vi "LoadWaferImg.vi"(8 "error in (no error)":errorcluster, 11 "FrontPanelData.lvclass":refnum<class "EpiWrapper.lvclass">) -> (0 "error out":errorcluster, 3 "FrontPanelData out":refnum<class "EpiWrapper.lvclass">)   [LabVIEW 2012]
uses:
  Classes/EpiWrapper.lvclass
  Controls/Waferimage.ctl
  Classes/EpiWrapper.lvclass/EpiWrapper.ctl
  Classes/Get_WaferImg.vi
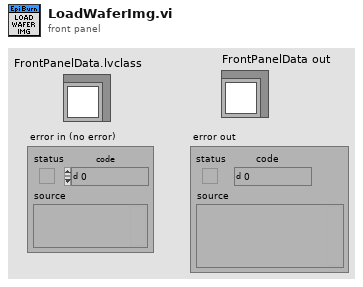
[diagram p1: front panel]
types:
  T1 = typedef "Waferimage.ctl" = picture
  T2 = typedef "LVBoundsTypeDef.ctl" = cluster{"Width":u32, "Height":u32}
  T3 = typedef "imagedata.ctl" = cluster{"image type":i32, "image depth":i32, "image":u8[], "mask":u8[], "colors":u32[], "Rectangle":cluster{"left":i16, "top":i16, "right":i16, "bottom":i16}}
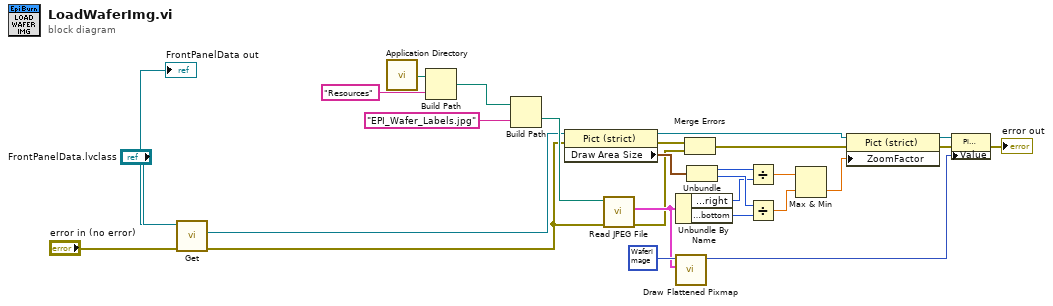
[diagram p0: block diagram]
diagram:
  n1 = call-poly "Get.vi"("error in (no error)"="error in (no error)", "FrontPanelData in"="FrontPanelData.lvclass") -> ("error out"=w2:errorcluster, "Wafer"=w3:refnum<vi>, "FrontPanelData out"=→"FrontPanelData out":refnum<class "EpiWrapper.lvclass">)  [unwired: 7 in]
  n2 = call <vilib>:"Application Directory.vi"() -> ("Application Directory"=w27:path)
  n3 = Build Path(base path=w27, name or relative path="Resources") -> (appended path=w8:path)
  n4 = Build Path(base path=w8, name or relative path="EPI_Wafer_Labels.jpg") -> (appended path=w6:path)
  n5 = property class="Pict (strict)"(reference=w3, error in=w2) -> (reference out=w17:refnum<vi>, error out=w14:errorcluster, "Draw Area Size"=w18:T2)
  n6 = call <vilib>:"Read JPEG File.vi"("error in (no error)"=w2, "path to JPEG file"=w6) -> ("error out"=w15:errorcluster, "image data"=w26:T3)  [unwired: 7 in, 1 out]
  n7 = Unbundle By Name(w26) -> ("Rectangle.right"=w22:i16, "Rectangle.bottom"=w23:i16)
  n8 = call <vilib>:"Draw Flattened Pixmap.vi"("image data"=w26, "picture"=T1 bytes[544710] ("Wafer")) -> ("new picture"=w19:picture)  [unwired: 7 in]
  n9 = Merge Errors(w14, w15) -> (w13:errorcluster)
  n10 = Unbundle(w18) -> ("Width"=w25:u32, "Height"=w24:u32)
  n11 = Divide(x=w25, y=w22) -> (x/y=w21:dbl)
  n12 = Divide(x=w24, y=w23) -> (x/y=w20:dbl)
  n13 = Max & Min(x=w21, y=w20) -> (min(x,y)=w16:dbl)  [unwired: 1 out]
  n14 = property class="Pict (strict)"(reference=w17, error in=w13, "ZoomFactor"=w16) -> (reference out=w12:refnum<vi>, error out=w11:errorcluster)
  n15 = property class="Pict (strict)"(reference=w12, error in=w11, "Value"=w19) -> (error out=→"error out":errorcluster)  [unwired: 1 out]
